vi "PROJECTE OCELL versió 0.1.vi"() -> ()   [LabVIEW 2020]
uses:
  <vilib>/numeric/Random Number (Range) DBL.vi
  <vilib>/MakerHub/LINX/Public/Utilities/Open Serial.vi
  <vilib>/MakerHub/LINX/LMH-LINX.lvlib
  <vilib>/MakerHub/LINX/Public/Sensors/Distance/Ultrasonic/Ultrasonic.lvlib
panel:
  out "appended array":cluster{i32[], dbl[]}[](array[cluster])
  in  "Velocitat de moviment":u32=100
  out "Error Out":errorcluster
  in  "Control d'aturada":bool
  in  "DI Channel":u8
  out "Device Name":string
  in  "Error In":errorcluster
  in  "Baud Rate Override":u32=9600
  in  "Serial Port":refnum<visa-resource-name>="N/A"
  out "Monitor":cluster{i32[], i64[]}[](graph)
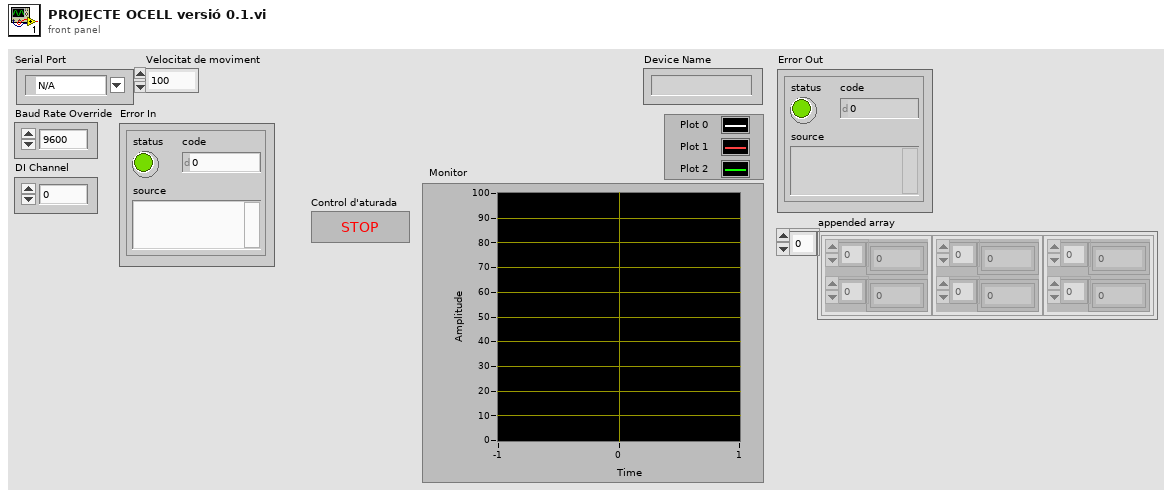
[diagram p1: front panel]
types:
  T1 = typedef "LMH-LINX.lvlib/LINX Ref.ctl" = cluster{"IO":T2, "Interface":T3, "LINX Device Config":T4}
  T2 = typedef "LMH-LINX.lvlib/Platform.ctl" = enum16{"Remote", "Local"}
  T3 = typedef "LMH-LINX.lvlib/Interface.ctl" = enum16{"Serial", "TCP"}
  T4 = typedef "LMH-LINX.lvlib/Device.lvlib/LINX Device Config.ctl" = cluster{"Interface":T3, "COM Port":refnum<visa-resource-name>, "TCP Configuration":T5, "Device Family":u8, "Device ID":u8, "Device Name":string, "TCP Ref":refnum<k5>, "Channels":T6}
  T5 = typedef "LMH-LINX.lvlib/Device.lvlib/TCP Config.ctl" = cluster{"IP Address":string, "Port":u16}
  T6 = typedef "LMH-LINX.lvlib/Channels.ctl" = cluster{"DI":u8[], "DO":u8[], "AI":u8[], "AO":u8[], "PWM":u8[], "QE":u8[], "UART":u8[], "I2C 2":u8[], "SPI":u8[], "CAN":u8[], "Servo":u8[], "AI Ref (V)":dbl, "AI Resolution (Bits)":u8, "AO Ref (V)":dbl, "AO Resolution (Bits)":u8}
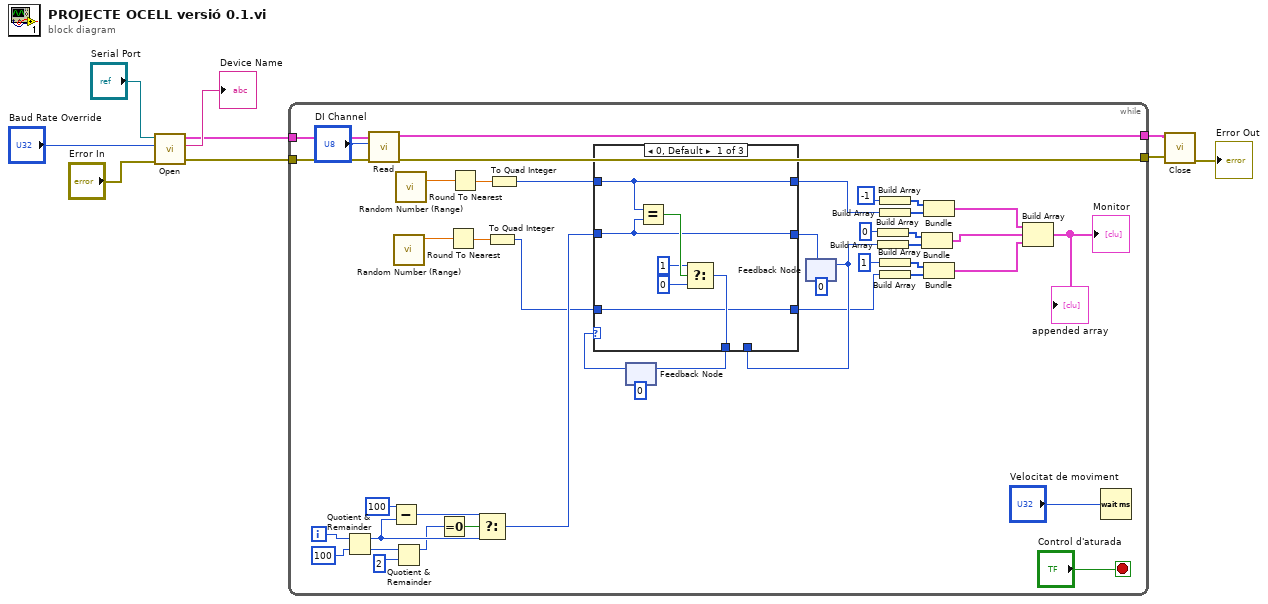
[diagram p0: block diagram]
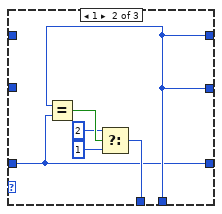
[diagram p2: hidden frame]
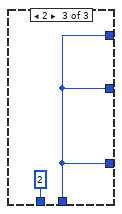
[diagram p3: hidden frame]
diagram:
  n1 = call-poly <vilib>:"Open.vi"("Error In"="Error In", "Baud Rate Override"="Baud Rate Override", "Serial Port"="Serial Port") -> ("Error Out"=w5:errorcluster, "Device Name"=→"Device Name":string, "LINX Resource"=w6:T1)  [unwired: 6 in]
  n2 = while {
    tunnel: w6 -> [w53]
    tunnel: w5 -> [w52]
    tunnel: [w45] -> w4
    tunnel: [w44] -> w3
    i -> [w34]
    stop <- "Control d'aturada" stop-if-true
    n3 = Quotient & Remainder(x=w34, y=100) -> (x-y*floor(x/y)=w31:i32, floor(x/y)=w28:i32)
    n4 = call <vilib>:"Read.vi"("Error In"=w52, "DI Channel"="DI Channel", "LINX Resource"=w53) -> ("Error Out"=w44:errorcluster, "LINX Resource"=w45:T1)  [unwired: 5 in, 2 out]
    n5 = Subtract(x=100 ("y"), y=w31) -> (x-y=w30:i32)
    n6 = call-poly <vilib>:"Random Number (Range).vi"() -> ("number"=w18:dbl)  [unwired: 11 in]
    n7 = Quotient & Remainder(x=w28, y=2) -> (x-y*floor(x/y)=w26:i32)  [unwired: 1 out]
    n8 = call-poly <vilib>:"Random Number (Range).vi"() -> ("number"=w25:dbl)  [unwired: 11 in]
    n9 = Equal To 0?(x=w26) -> (x = 0?=w27:bool)
    n10 = Round To Nearest(number=w18) -> (nearest integer value=w19:dbl)
    n11 = Round To Nearest(number=w25) -> (nearest integer value=w24:dbl)
    n12 = Select(t=w30, s=w27, f=w31) -> (s? t:f=w20:i32)
    n13 = To Quad Integer(1:w19) -> (0:w14:i64)
    n14 = To Quad Integer(1:w24) -> (0:w23:i64)
    n15 = feedback #1(0 ("f")) -> (w11:i32)
    n16 = feedback #2(0) -> (w16:i32)
    n17 = case shown="0, Default" w11 {
      tunnel: w23 -> [w60 _ _]
      tunnel: [w60 w62 w67] -> w22
      tunnel: w20 -> [w57 _ _]
      tunnel: [w57 w62 w67] -> w17
      tunnel: w16 -> [_ w62 w67]
      tunnel: w14 -> [w55 w61 _]
      tunnel: [w55 w61 w67] -> w13
      tunnel: [w58 w63 2 ("f")] -> w12
      frame 0, Default {
        n18 = Equal?(x=w60, y=w57) -> (x = y?=w59:bool)
        n19 = Select(t=1, s=w59, f=0) -> (s? t:f=w58:i32)
      }
      frame 1 {
        n20 = Equal?(x=w62, y=w61) -> (x = y?=w66:bool)
        n21 = Select(t=2, s=w66, f=1) -> (s? t:f=w63:i32)
      }
      frame 2 {
      }
    }
    n22 = feedback-in #1(w12) -> ()
    n23 = feedback-in #2(w17) -> ()
    n24 = Build Array(0) -> (w38:i32[])
    n25 = Build Array(w16) -> (w21:i32[])
    n26 = Build Array(-1) -> (w40:i32[])
    n27 = Build Array(w22) -> (w41:i64[])
    n28 = Build Array(1) -> (w36:i32[])
    n29 = Build Array(w13) -> (w35:i64[])
    n30 = Bundle(w38, w21) -> (w48:cluster{i32[], i32[]})  [unwired: 1 in]
    n31 = Bundle(w40, w41) -> (w49:cluster{i32[], i64[]})  [unwired: 1 in]
    n32 = Bundle(w36, w35) -> (w47:cluster{i32[], i64[]})  [unwired: 1 in]
    n33 = Build Array(w49, w48, w47) -> (→"Monitor" →"appended array":cluster{i32[], i64[]}[])
    n34 = Wait (ms)(milliseconds to wait="Velocitat de moviment") -> ()  [unwired: 1 out]
  }
  n35 = call <vilib>:"Close.vi"("Error In"=w3, "LINX Resource"=w4) -> ("Error Out"=→"Error Out":errorcluster)  [unwired: 9 in]
